vi "AddPerformancePropertiesToSpeedProfile.vi"(6 "Speed Profile":dbl[](array[numeric]), 8 "error in (no error)":errorcluster, 9 "Channel":string, 10 "Group":string, 11 "Tdms Ref":refnum<k34>) -> (0 "error out":errorcluster, 1 "Channel out":string, 2 "Group out":string, 3 "Tdms Ref out":refnum<k34>)   [LabVIEW 2017, in "DataExplorerSupport.lvlib"]
uses:
  <vilib>/addons/InsightCM/Utilities/DataExplorerSupport/DataExplorerSupport.lvlib
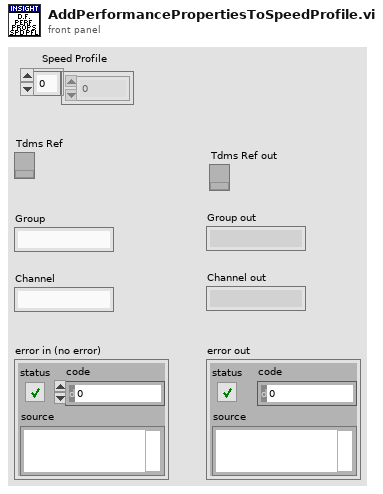
[diagram p1: front panel]
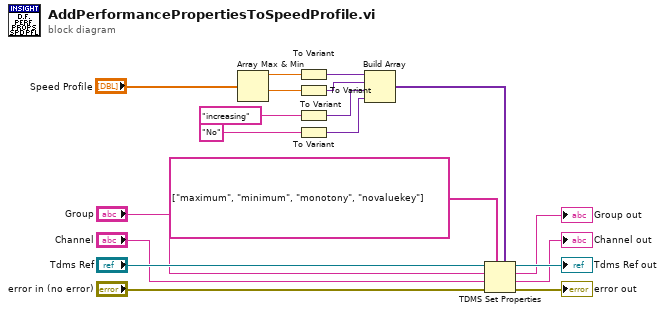
[diagram p0: block diagram]
diagram:
  n1 = Array Max & Min(array="Speed Profile") -> (max value=w18:dbl, min value=w16:dbl)  [unwired: 2 out]
  n2 = To Variant(anything=w18) -> (Variant=w17:variant)
  n3 = To Variant(anything=w16) -> (Variant=w15:variant)
  n4 = To Variant(anything="increasing") -> (Variant=w13:variant)
  n5 = To Variant(anything="No") -> (Variant=w11:variant)
  n6 = Build Array(w17, w15, w13, w11) -> (w10:variant[])
  n7 = TDMS Set Properties(5:w10, 7:string[] ["maximum", "minimum", "monotony", "novaluekey"] ("property names"), 8:"error in (no error)", 9:"Channel", 10:"Group", 11:"Tdms Ref") -> (0:→"error out":errorcluster, 1:→"Channel out":string, 2:→"Group out":string, 3:→"Tdms Ref out":refnum<k34>)
